vi "CICLOS_ANIDADOS.vi"() -> ()   [LabVIEW 2013]
panel:
  out "Contador":dbl
  out "Número 50-100":dbl
  # "GENERAR 10 NÚMEROS ENTRE 50-150, USAR UN CICLO WHILE\nPARA VALIDAR QUE EL NÚMERO SE ENCUENTRE EN ESE RANGO ANTES DE \nPRESENTARLOS\nIR CONTANDO LOS NÚMEROS."
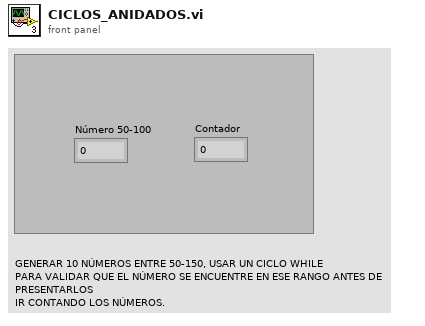
[diagram p1: front panel]
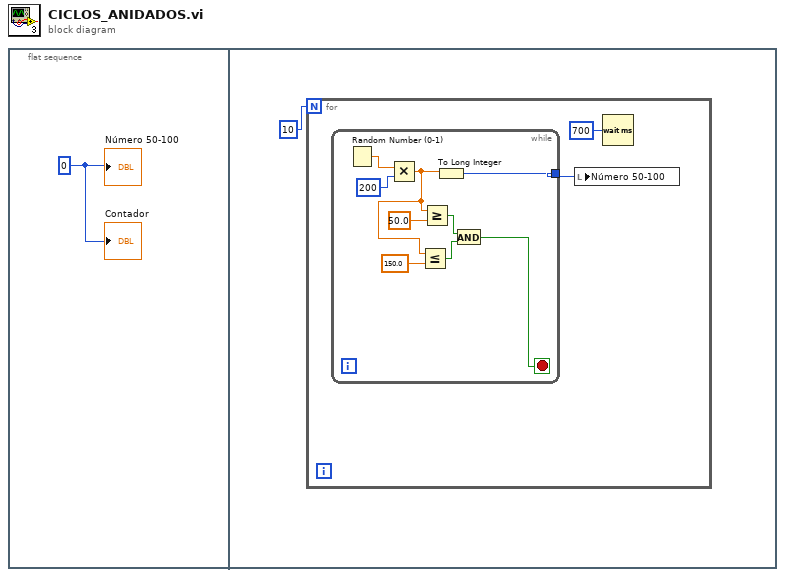
[diagram p0: block diagram]
diagram:
  n1 = flat-sequence {
    frame #0 {
      w1 = 0
      "Número 50-100" <- w1
      "Contador" <- w1
    }
    frame #1 {
      n2 = for {
        N: 10 -> [_]
        n3 = while {
          tunnel: [w11] -> w4
          stop <- w5 stop-if-true
          n4 = Random Number (0-1)() -> (number: 0 to 1=w13:dbl)
          n5 = Multiply(x=w13, y=200) -> (x*y=w8:dbl)
          n6 = Less Or Equal?(x=w8, y=150.0) -> (x <= y?=w6:bool)
          n7 = Greater Or Equal?(x=w8, y=50.0) -> (x >= y?=w7:bool)
          n8 = To Long Integer(number=w8) -> (32bit integer=w11:i32)
          n9 = And(x=w7, y=w6) -> (x .and. y?=w5:bool)
        }
        n10 = local write "Número 50-100"(w4) -> ()
        n11 = Wait (ms)(milliseconds to wait=u32 700) -> ()  [unwired: 1 out]
      }
    }
  }
